vi "BIO_set_SSL_mode.vi"(8 "error in (no error)":errorcluster, 10 "Client?":bool, 11 "BIO in":refnum<class "BIO.lvclass">) -> (0 "error out":errorcluster, 3 "BIO out":refnum<class "BIO.lvclass">)   [LabVIEW 2013, in "SSL_Lib.lvlib" / "BIO.lvclass"]
uses:
  BIO.lvclass
  SSL-Lib/SSL-Lib.lvclass/SSL-Lib.ctl
  BIO.lvclass/BIO.ctl
  SSL-Lib/Read Crypto Library Path.vi
  Read Handle.vi
  SSL-Lib/SSL-Lib.lvclass
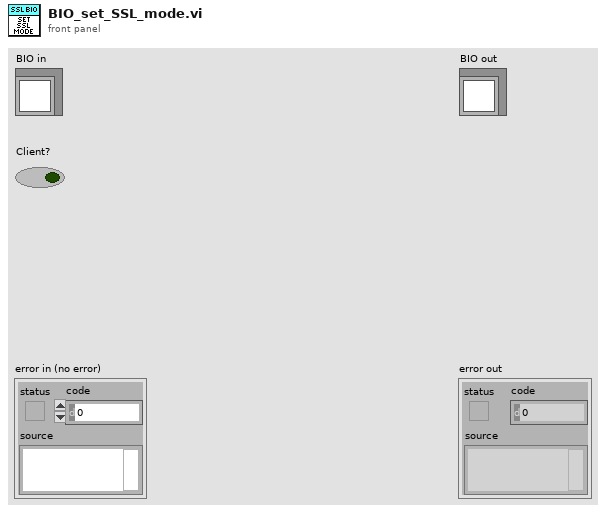
[diagram p1: front panel]
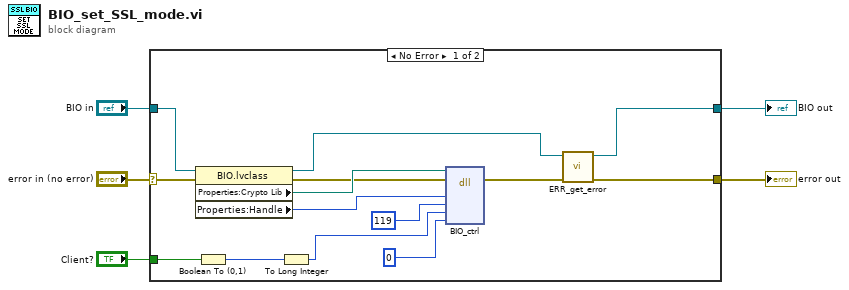
[diagram p0: block diagram]
diagram:
  n1 = case shown="No Error" "error in (no error)" {
    selector: "error in (no error)" -> [w18 w21]
    tunnel: [w12 w21] -> w4
    tunnel: [w10 w20] -> w2
    tunnel: "BIO in" -> [w17 w20]
    tunnel: "Client?" -> [w9 _]
    frame No Error {
      n2 = property class="BIO.lvclass"(reference=w17, error in=w18) -> (reference out=w11:refnum<class "BIO.lvclass">, error out=w14:errorcluster, "Properties:Crypto Lib"=w15:path, "Properties:Handle"=w16:u64)
      n3 = Boolean To (0,1)(Boolean=w9) -> (0, 1=w8:i16)
      n4 = To Long Integer(number=w8) -> (32bit integer=w7:i32)
      n5 = dll-call lib="C:/Program Files (x86)/National Instruments/Shared/nissl/NIlibeay32.dll" fn="BIO_ctrl"(path in=w15, error in=w14, "BIO"=w16, "cmd"=119, "larg"=w7, "parg"=0 ("larg")) -> (error out=w13:errorcluster)  [unwired: 6 in, 1 out]
      n6 = call "ERR_get_error.vi"("error in (no error)"=w13, "SSL-Lib in"=w11) -> ("error out"=w12:errorcluster, "SSL-Lib out"=w10:refnum<class "BIO.lvclass">)  [unwired: 8 in]
    }
    frame Error {
    }
  }
  "error out" <- w4
  "BIO out" <- w2
